vi "Icon_Count blank rows columns.vi"(8 "Error":errorcluster, 9 "Near (f)\nfar (t)":bool, 10 "Height (f)\nWidth (t)":bool, 11 "2D Image":T1) -> (0 "Error Out":errorcluster, 1 "Blank Row count":i32, 3 "Last Index Out":i32)   [LabVIEW 2009]
uses:
  Controls/Array/Color Box Array_2D Icon Viewer.ctl
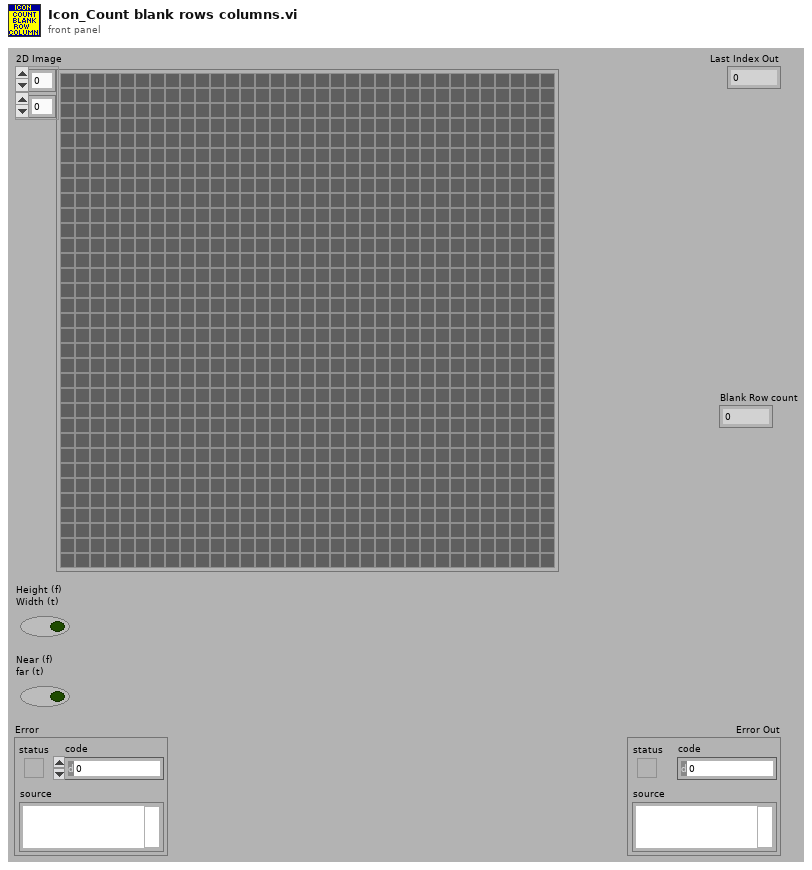
[diagram p1: front panel]
types:
  T1 = typedef "Color Box Array_2D Icon Viewer.ctl" = u32[][]
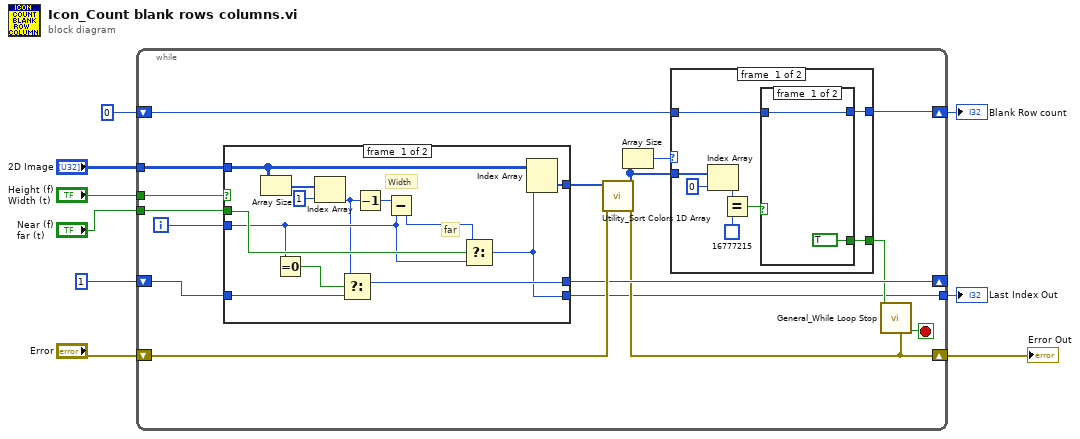
[diagram p0: block diagram]
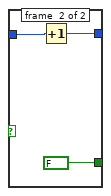
[diagram p2: hidden frame]
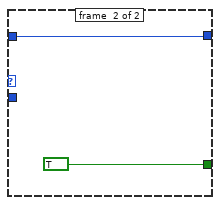
[diagram p3: hidden frame]
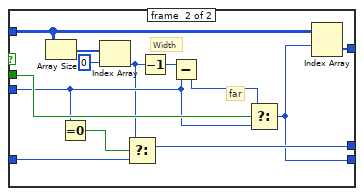
[diagram p4: hidden frame]
diagram:
  n1 = while {
    tunnel: "2D Image" -> [w22]
    tunnel: "Height (f)\nWidth (t)" -> [w25]
    tunnel: "Near (f)\nfar (t)" -> [w24]
    shift-right: [w15] -> w8
    shift-left: "Error" -> [w20]
    shift-right: [w18] -> _
    shift-left: 1 -> [w17]
    tunnel: [w12] -> w3
    shift-right: [w10] -> w1
    shift-left: 0 ("Last Index Out") -> [w11]
    i -> [w23]
    stop <- w16 stop-if-true
    n2 = case shown="True" w25 {
      tunnel: w24 -> [w48 w61]
      tunnel: w23 -> [w46 w59]
      tunnel: w22 -> [w53 w66]
      tunnel: [w52 w65] -> w21
      tunnel: [w43 w56] -> w18
      tunnel: w17 -> [w42 w55]
      tunnel: [w41 w54] -> w12
      frame #0 {
        # "far"
        # "Width"
        n3 = Array Size(array=w53) -> (size(s)=w51:i32[])
        n4 = Equal To 0?(x=w46) -> (x = 0?=w45:bool)
        n5 = Index Array(array=w51, index=1) -> (element=w44:i32)
        n6 = Select(t=w44, s=w45, f=w42) -> (s? t:f=w43:i32)
        n7 = Decrement(x=w44) -> (x-1=w49:i32)
        n8 = Subtract(x=w49, y=w46) -> (x-y=w47:i32)
        n9 = Select(t=w47, s=w48, f=w46) -> (s? t:f=w41:i32)
        n10 = Index Array(array=w53, index (col)=w41) -> (element=w52:u32[])  [unwired: 1 in]
      }
      frame #1 {
        # "far"
        # "Width"
        n11 = Array Size(array=w66) -> (size(s)=w64:i32[])
        n12 = Equal To 0?(x=w59) -> (x = 0?=w58:bool)
        n13 = Index Array(array=w64, index=0) -> (element=w57:i32)
        n14 = Select(t=w57, s=w58, f=w55) -> (s? t:f=w56:i32)
        n15 = Decrement(x=w57) -> (x-1=w62:i32)
        n16 = Subtract(x=w62, y=w59) -> (x-y=w60:i32)
        n17 = Select(t=w60, s=w61, f=w59) -> (s? t:f=w54:i32)
        n18 = Index Array(array=w66, index (row)=w54) -> (element=w65:u32[])  [unwired: 1 in]
      }
    }
    n19 = call "Utility_Sort Colors 1D Array.vi"("Error"=w20, "Colors"=w21) -> ("Error Out"=w15:errorcluster, "Sorted By Quantity Out"=w13:u32[])  [unwired: 7 in, 1 out]
    n20 = Array Size(array=w13) -> (size(s)=w19:i32)
    n21 = case shown="1" w19 {
      tunnel: [w28 TRUE] -> w14
      tunnel: w13 -> [w33 _]
      tunnel: w11 -> [w27 w39]
      tunnel: [w26 w39] -> w10
      frame #0 {
        n22 = Index Array(array=w33, index=0) -> (element=w31:u32)
        n23 = Equal?(x=w31, y=u32 16777215) -> (x = y?=w29:bool)
        n24 = case shown="False" w29 {
          tunnel: [TRUE FALSE] -> w28
          tunnel: w27 -> [w34 w37]
          tunnel: [w34 w36] -> w26
          frame #0 {
          }
          frame #1 {
            n25 = Increment(x=w37) -> (x+1=w36:i32)
          }
        }
      }
      frame #1 {
      }
    }
    n26 = call "General_While Loop Stop.vi"("Error In"=w15, "Stop 1 In"=w14) -> ("Stop Out3"=w16:bool)  [unwired: 5 in, 3 out]
  }
  "Error Out" <- w8
  "Last Index Out" <- w3
  "Blank Row count" <- w1
